vi "ClientPool_GetClients_ClientsCreatedWithNonZeroGrpcId.vi"(8 "error in (no error)":errorcluster) -> (0 "error out":errorcluster, 2 "result":string, 3 "pass":bool)   [LabVIEW 2020, in "MeasurementServerTests.lvlib"]
uses:
  MeasurementServerTests.lvlib
  Runtime/MeasurementLink Measurement Server/Classes/GrpcClientPool/GrpcClientPool.lvclass
  Runtime/MeasurementLink Measurement Server/Classes/GrpcClientPool/FGV Action.ctl
panel:
  in  "Action":T1
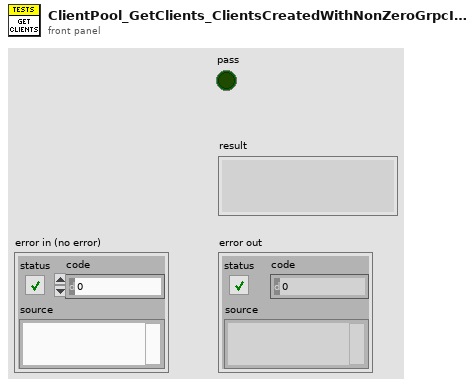
[diagram p1: front panel]
types:
  T1 = typedef "gRPC Utilities.lvlib/GrpcClientPool.lvclass/FGV Action.ctl" = enum16{"Get Discovery Client", "Get Session Client", "Get Pinmap Client", "Destroy Clients"}
  T2 = typedef "grpc-lvsupport-release.lvlib/grpcId.ctl" = u64
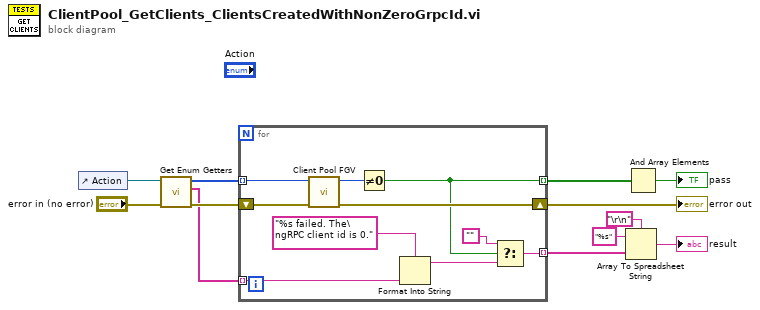
[diagram p0: block diagram]
diagram:
  n1 = control-ref of="Action"() -> (w1:refnum<vi>)
  n2 = call "Get Enum Getters.vi"("error in (no error)"="error in (no error)", "enum ref in"=w1) -> ("error out"=w5:errorcluster, "enum strings"=w4:string[], "enum numbers"=w3:i32[])  [unwired: 7 in]
  n3 = for {
    shift-right: [w21] -> w12
    shift-left: w5 -> [w22]
    tunnel: w3 -> [w13] mode=indexing
    tunnel: [w18] -> w11 mode=indexing
    tunnel: w4 -> [w20] mode=indexing
    tunnel: [w15] -> w9 mode=indexing
    n4 = call "Client Pool FGV.vi"("error in (no error)"=w22, "Action"=w13) -> ("error out"=w21:errorcluster, "grpc client id"=w14:T2)  [unwired: 8 in]
    n5 = Not Equal To 0?(x=w14) -> (x != 0?=w18:bool)
    n6 = Format Into String(format string="%s failed. The\ngRPC client id is 0." ("result"), w20) -> (resulting string=w17:string)  [unwired: 2 in, 1 out]
    n7 = Select(t="", s=w18, f=w17) -> (s? t:f=w15:string)
  }
  "error out" <- w12
  n8 = Array To Spreadsheet String(delimiter (Tab)="\r\n", array=w9, 3:"%s" ("format string")) -> (spreadsheet string=→"result":string)
  n9 = And Array Elements(Boolean array=w11) -> (logical AND=→"pass":bool)
